vi "Inficon - Set parameter.vi"(8 "Error In":errorcluster, 9 "Param value":string, 10 "Param number":u8 max=99 step=1, 11 "COM in":refnum<visa-resource-name>) -> (0 "Error Out":errorcluster, 3 "COM out":refnum<visa-resource-name>)   [LabVIEW 2014]
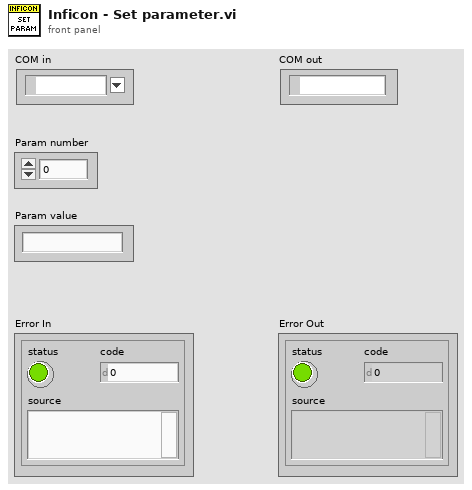
[diagram p1: front panel]
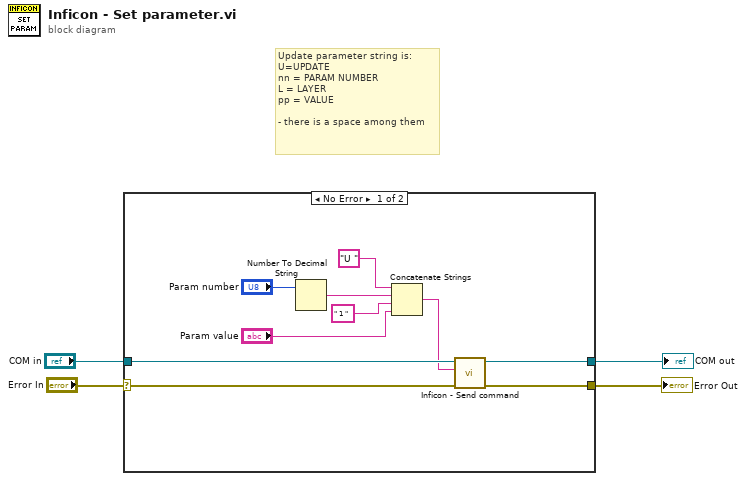
[diagram p0: block diagram]
diagram:
  # "Update parameter string is:\nU=UPDATE\nnn = PARAM NUMBER\nL = LAYER\npp = VALUE\n\n- there is a space among them"
  n1 = case shown="No Error" "Error In" {
    selector: "Error In" -> [w14 w16]
    tunnel: [w13 w16] -> w3
    tunnel: "COM in" -> [w12 w15]
    tunnel: [w11 w15] -> w1
    frame No Error {
      n2 = Number To Decimal String(number="Param number") -> (decimal integer string=w8:string)  [unwired: 1 in]
      n3 = Concatenate Strings("U ", w8, " 1 ", "Param value") -> (w5:string)
      n4 = call "Inficon - Send command.vi"("Error In"=w14, "Command"=w5, "COM in"=w12) -> ("Error Out"=w13:errorcluster, "COM out"=w11:refnum<visa-resource-name>)  [unwired: 6 in, 1 out]
    }
    frame Error {
    }
  }
  "COM out" <- w1
  "Error Out" <- w3
